vi "ScanFeedback.vi"(2 "measurement type":T1(tab)) -> (1 "V breakdown":dbl, 5 "V depletion":dbl, 6 "Maximum current fluctuations [%]":dbl[](array[numeric]), 8 "Ris [MOhm]":dbl, 9 "Cis @300V [pF/cm]":dbl)   [LabVIEW 2013]
uses:
  globals/QC_MeasurementSetup.vi
  <vilib>/Analysis/NI_AALPro.lvlib
  <vilib>/Analysis/NI_AALBase.lvlib
panel:
  out "MEAN":dbl
  out "STD":dbl
  out "Index lin fit 1":dbl
  out "Slope":dbl
  out "capSquare1":dbl[](array[numeric])
  out "volts1":dbl[](array[numeric])
  out "volts2":dbl[](array[numeric])
  out "capSquare2":dbl[](array[numeric])
  out "deriv":dbl[](array[numeric])
  out "Slope 2":dbl
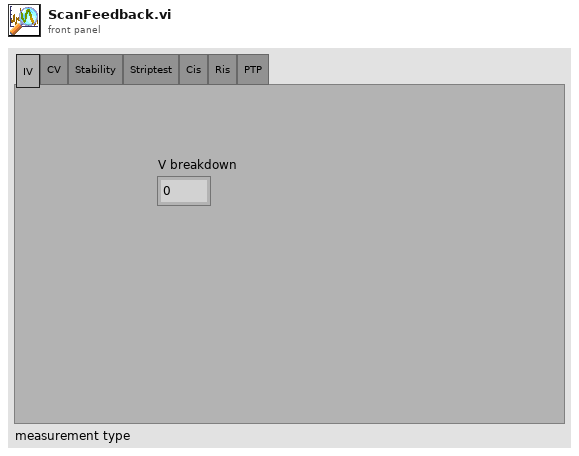
[diagram p1: front panel]
types:
  T1 = enum32{"IV", "CV", "Stability", "Striptest", "Cis", "Ris", "PTP"}
  T2 = enum16{"Reset", "Read Array", "Read Element", "Write Element", "Write Array", "Add Element", "Add Array"}
  T3 = cluster{"Supply":refnum<class "SupplyControl.lvclass">, "Arduino":refnum<class "ArduinoControl.lvclass">, "Measurement switch":refnum<class "Switching.lvclass">, "Initial Voltage [V]":dbl, "Final Voltage [V]":dbl, "Step Size [V]":dbl, "Step Interval [s]":i32, "Number Of Steps":u32, "Ramp down steps [V]":dbl, "Ramp down Interval [s]":i32, "hold steps":i32, "Set Current Limit?":bool, "Current Limit [µA]":dbl, "Temperature Readout":enum16{"Read Arduino", "Enter manually"}, "Supply Name":string, "V_breakdown Limit [V]":dbl, "Measurement switch used?":bool}
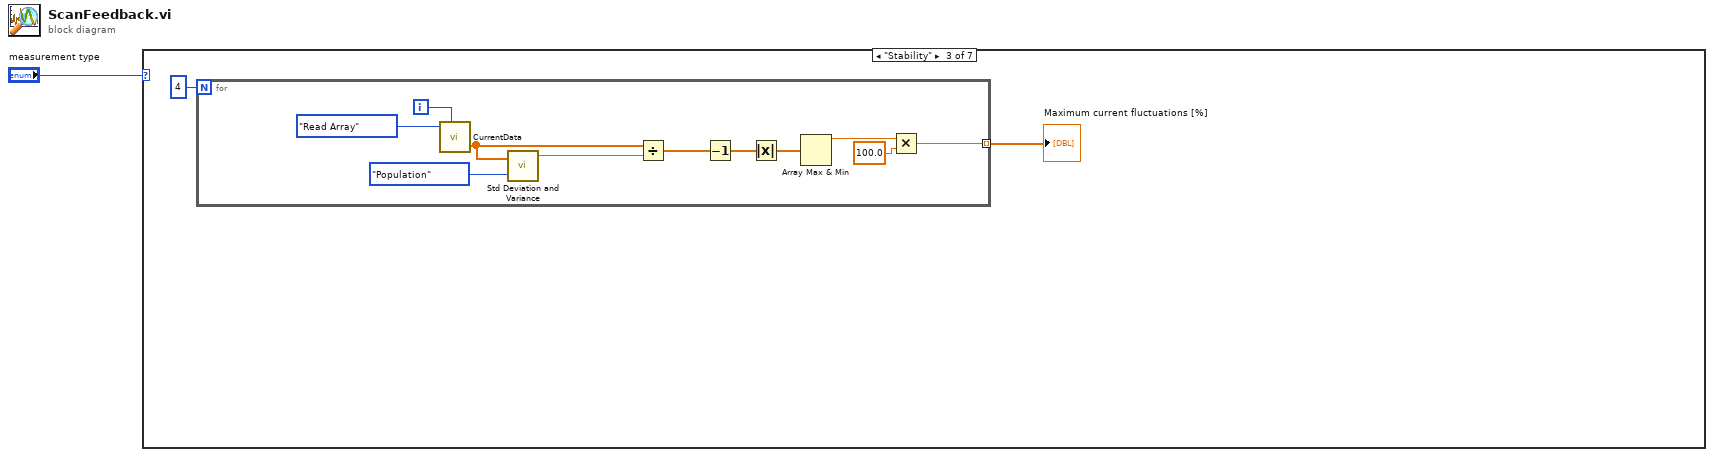
[diagram p0: block diagram]
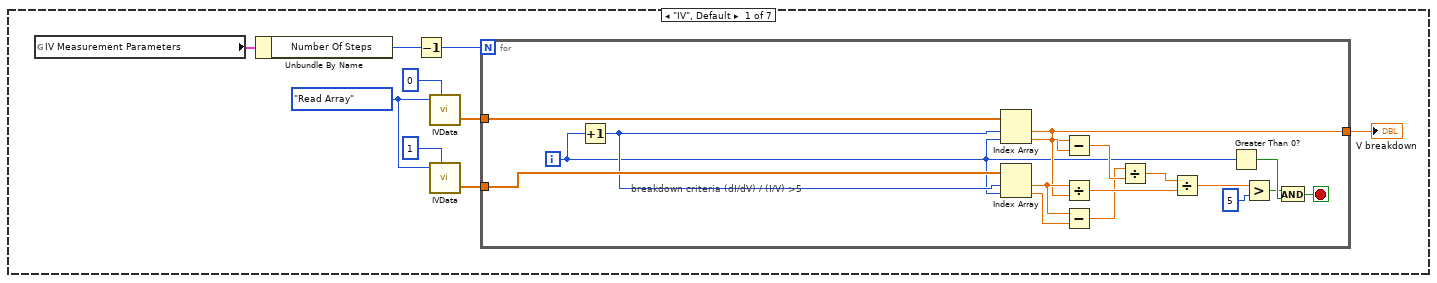
[diagram p2: hidden frame]
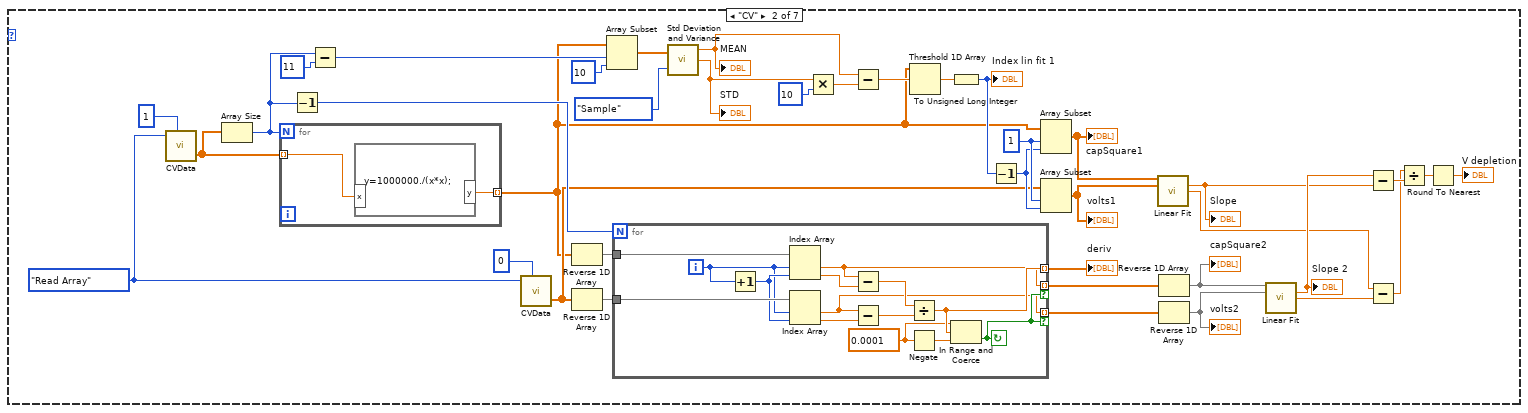
[diagram p3: hidden frame]
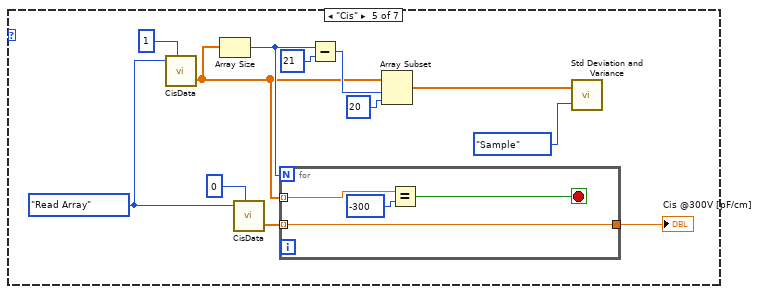
[diagram p5: hidden frame]
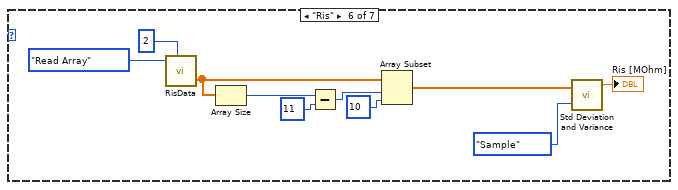
[diagram p6: hidden frame]
diagram:
  n1 = case shown="\"Stability\"" "measurement type" {
    frame "IV", Default {
      w8 = T2."Read Array" ("Action")
      n2 = global read "QC_MeasurementSetup.vi" "IV Measurement Parameters"() -> (w3:T3)
      n3 = Unbundle By Name(w3) -> ("Number Of Steps"=w2:u32)
      n4 = Decrement(x=w2) -> (x-1=w5:u32)
      n5 = call "IVData.vi"("Action"=w8, "Array No."=0) -> ("Array OUT"=w6:dbl[])  [unwired: 3 in, 1 out]
      n6 = call "IVData.vi"("Action"=w8, "Array No."=1) -> ("Array OUT"=w7:dbl[])  [unwired: 3 in, 1 out]
      n7 = for {
        N: w5 -> [_]
        tunnel: w6 -> [w26]
        tunnel: w7 -> [w27]
        tunnel: [w15] -> w4
        i -> [w13]
        stop <- w11 stop-if-true
        # "breakdown criteria (dI/dV) / (I/V) >5"
        n8 = Increment(x=w13) -> (x+1=w23:i32)
        n9 = Index Array(array=w26, index #1=w23, index #2=w13) -> (element #1=w15:dbl, element #2=w25:dbl)
        n10 = Index Array(array=w27, index #1=w23, index #2=w13) -> (element #1=w18:dbl, element #2=w24:dbl)
        n11 = Subtract(x=w15, y=w25) -> (x-y=w20:dbl)
        n12 = Divide(x=w18, y=w15) -> (x/y=w21:dbl)
        n13 = Subtract(x=w18, y=w24) -> (x-y=w19:dbl)
        n14 = Divide(x=w19, y=w20) -> (x/y=w22:dbl)
        n15 = Divide(x=w22, y=w21) -> (x/y=w16:dbl)
        n16 = Greater Than 0?(x=w13) -> (x > 0?=w14:bool)
        n17 = Greater?(x=w16, y=5) -> (0:w12:bool)
        n18 = And(x=w12, y=w14) -> (x .and. y?=w11:bool)
      }
      "V breakdown" <- w4
    }
    frame "CV" {
      w38 = T2."Read Array" ("Action")
      w35 = 1
      n19 = call "CVData.vi"("Action"=w38, "Array No."=1) -> ("Array OUT"=w29:dbl[])  [unwired: 3 in, 1 out]
      n20 = Array Size(array=w29) -> (size(s)=w30:i32)
      n21 = for {
        N: w30 -> [_]
        tunnel: w29 -> [w68] mode=indexing
        tunnel: [w67] -> w28 mode=indexing
        n22 = formula code="y=1000000./(x*x);"("x"=w68) -> ("y"=w67:dbl)
      }
      n23 = Decrement(x=w30) -> (x-1=w51:i32)
      n24 = Subtract(x=w30, y=11) -> (x-y=w65:i32)
      n25 = call "CVData.vi"("Action"=w38, "Array No."=0) -> ("Array OUT"=w32:dbl[])  [unwired: 3 in, 1 out]
      n26 = Reverse 1D Array(array=w28) -> (reversed array=w54:dbl[])
      n27 = Reverse 1D Array(array=w32) -> (reversed array=w31:dbl[])
      n28 = Array Subset(array=w28, index=w65, length=10) -> (w63:dbl[])
      n29 = for {
        N: w51 -> [_]
        tunnel: w54 -> [w82]
        tunnel: [w75] -> w53 mode=indexing if=w76
        tunnel: [w71] -> w50 mode=indexing if=w76
        tunnel: [w79] -> w47 mode=indexing
        tunnel: w31 -> [w74]
        i -> [w72]
        stop <- w76 continue-if-true
        w77 = 0.0001
        n30 = Increment(x=w72) -> (x+1=w73:i32)
        n31 = Index Array(array=w82, index #1=w72, index #2=w73) -> (element #1=w75:dbl, element #2=w80:dbl)
        n32 = Index Array(array=w74, index #1=w72, index #2=w73) -> (element #1=w71:dbl, element #2=w70:dbl)
        n33 = Subtract(x=w75, y=w80) -> (x-y=w81:dbl)
        n34 = Subtract(x=w71, y=w70) -> (x-y=w69:dbl)
        n35 = Divide(x=w81, y=w69) -> (x/y=w79:dbl)
        n36 = Negate(x=w77) -> (-x=w78:dbl)
        n37 = In Range and Coerce(upper limit=w77, x=w79, lower limit=w78) -> (In Range?=w76:bool)  [unwired: 1 out]
      }
      "deriv" <- w47
      n38 = call <vilib>:"Std Deviation and Variance.vi"("X"=w63, "Weighting (Sample)"=enum16{"Sample", "Population"}."Sample") -> ("mean"=w59:dbl, "standard deviation"=w48:dbl)  [unwired: 1 out]
      "MEAN" <- w59
      "STD" <- w48
      n39 = Multiply(x=w48, y=10) -> (x*y=w60:dbl)
      n40 = Subtract(x=w59, y=w60) -> (x-y=w58:dbl)
      n41 = Threshold 1D Array(2:w58, 3:w28) -> (0:w57:dbl)  [unwired: 1 in]
      n42 = To Unsigned Long Integer(number=w57) -> (unsigned 32bit integer=w56:u32)
      "Index lin fit 1" <- w56
      n43 = Decrement(x=w56) -> (x-1=w34:u32)
      n44 = Array Subset(array=w28, index=w35, length=w34) -> (w55:dbl[])
      "capSquare1" <- w55
      n45 = Array Subset(array=w32, index=w35, length=w34) -> (w33:dbl[])
      "volts1" <- w33
      n46 = call <vilib>:"Linear Fit.vi"("Y"=w55, "X"=w33) -> ("slope"=w45:dbl, "intercept"=w43:dbl)  [unwired: 9 in, 3 out]
      "Slope" <- w45
      n47 = Reverse 1D Array(array=w53) -> (reversed array=w52:dbl[])
      "capSquare2" <- w52
      n48 = Reverse 1D Array(array=w50) -> (reversed array=w49:dbl[])
      "volts2" <- w49
      n49 = call <vilib>:"Linear Fit.vi"("Y"=w52, "X"=w49) -> ("slope"=w46:dbl, "intercept"=w44:dbl)  [unwired: 9 in, 3 out]
      "Slope 2" <- w46
      n50 = Subtract(x=w46, y=w45) -> (x-y=w42:dbl)
      n51 = Subtract(x=w43, y=w44) -> (x-y=w41:dbl)
      n52 = Divide(x=w41, y=w42) -> (x/y=w40:dbl)
      n53 = Round To Nearest(number=w40) -> (nearest integer value=→"V depletion":dbl)
    }
    frame "Stability" {
      n54 = for {
        N: 4 -> [_]
        tunnel: [w85] -> w83 mode=indexing
        i -> [w94]
        n55 = call "CurrentData.vi"("Action"=T2."Read Array", "Array No."=w94) -> ("Array OUT"=w91:dbl[])  [unwired: 3 in, 1 out]
        n56 = call <vilib>:"Std Deviation and Variance.vi"("X"=w91, "Weighting (Sample)"=enum16{"Sample", "Population"}."Population") -> ("mean"=w92:dbl)  [unwired: 2 out]
        n57 = Divide(x=w91, y=w92) -> (x/y=w90:dbl[])
        n58 = Decrement(x=w90) -> (x-1=w89:dbl[])
        n59 = Absolute Value(x=w89) -> (abs(x)=w88:dbl[])
        n60 = Array Max & Min(array=w88) -> (max value=w87:dbl)  [unwired: 3 out]
        n61 = Multiply(x=w87, y=100.0) -> (x*y=w85:dbl)
      }
      "Maximum current fluctuations [%]" <- w83
    }
    frame "Striptest" {
    }
    frame "Cis" {
      w101 = T2."Read Array" ("Action")
      n62 = call "CisData.vi"("Action"=w101, "Array No."=1) -> ("Array OUT"=w98:dbl[])  [unwired: 3 in, 1 out]
      n63 = Array Size(array=w98) -> (size(s)=w99:i32)
      n64 = call "CisData.vi"("Action"=w101, "Array No."=0) -> ("Array OUT"=w97:dbl[])  [unwired: 3 in, 1 out]
      n65 = for {
        N: w99 -> [_]
        tunnel: w98 -> [w110] mode=indexing
        tunnel: w97 -> [w108] mode=indexing
        tunnel: [w108] -> w96
        stop <- w109 stop-if-true
        n66 = Equal?(x=w110, y=-300) -> (x = y?=w109:bool)
      }
      "Cis @300V [pF/cm]" <- w96
      n67 = Subtract(x=w99, y=21) -> (x-y=w103:i32)
      n68 = Array Subset(array=w98, index=w103, length=20) -> (w102:dbl[])
      n69 = call <vilib>:"Std Deviation and Variance.vi"("X"=w102, "Weighting (Sample)"=enum16{"Sample", "Population"}."Sample") -> ()  [unwired: 3 out]
    }
    frame "Ris" {
      n70 = call "RisData.vi"("Action"=T2."Read Array", "Array No."=2) -> ("Array OUT"=w112:dbl[])  [unwired: 3 in, 1 out]
      n71 = Array Size(array=w112) -> (size(s)=w120:i32)
      n72 = Subtract(x=w120, y=11) -> (x-y=w117:i32)
      n73 = Array Subset(array=w112, index=w117, length=10) -> (w116:dbl[])
      n74 = call <vilib>:"Std Deviation and Variance.vi"("X"=w116, "Weighting (Sample)"=enum16{"Sample", "Population"}."Sample") -> ("mean"=→"Ris [MOhm]":dbl)  [unwired: 2 out]
    }
    frame "PTP" {
    }
  }
